vi "ReadIOValues b2g2.vi"(2 "error in":errorcluster, 3 "Output - Cluster b2g2 2":T1 {"TS-5 [°C]" format="%#.2g"; "pHS-1 [pH]" format="%.2g"; "TS-4 [°C]" format="%#.2g"; "FS-2 [l]" format="%.2g"; "FS-1 [l]" format="%.2g"; "DS-1 [bar]" format="%#.2g"; "DFS-1 [l/min]" format="%#.2g"; "FS-3 [l]" format="%.2g"; "DFS-1 [dl]" format="%.0g"}) -> (0 "error out":errorcluster, 1 "Output - Cluster b2g2":T1 {"TS-5 [°C]" format="%#.2g"; "pHS-1 [pH]" format="%.2g"; "TS-4 [°C]" format="%#.2g"; "FS-2 [l]" format="%.2g"; "FS-1 [l]" format="%.2g"; "DS-1 [bar]" format="%#.2g"; "DFS-1 [l/min]" format="%#.2g"; "FS-3 [l]" format="%.2g"; "DFS-1 [dl]" format="%.0g"})   [LabVIEW 2011]
uses:
  Output - Cluster b2g2.ctl
  <vilib>/functionblocks/Counter/Count Up/Count Up.vi
  <vilib>/functionblocks/FB Core/FB Core.xnode
  <vilib>/functionblocks/NI_FunctionBlock Libraries.lvlib
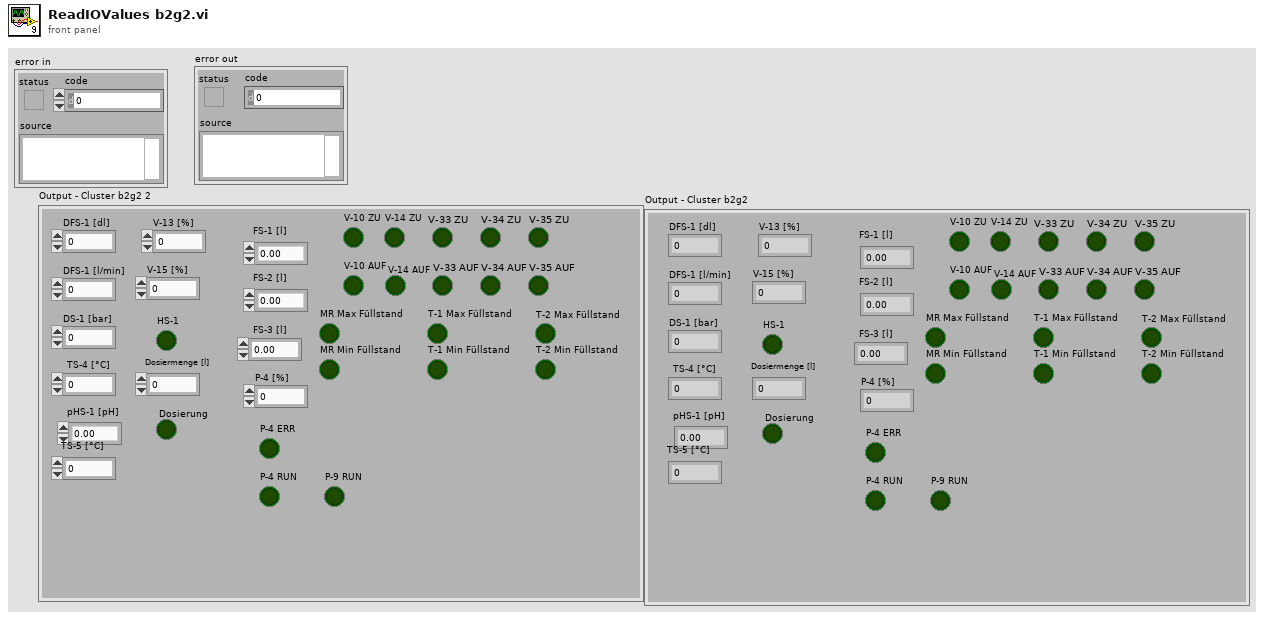
[diagram p1: front panel]
types:
  T1 = typedef "Output - Cluster b2g2.ctl" = cluster{"DFS-1 [dl]":u64, "FS-3 [l]":dbl, "DFS-1 [l/min]":dbl, "DS-1 [bar]":dbl, "V-10 ZU":bool, "V-14 ZU":bool, "FS-1 [l]":dbl, "FS-2 [l]":dbl, "TS-4 [°C]":dbl, "HS-1":bool, "V-13 [%]":u8, "V-15 [%]":u8, "P-4 [%]":u8, "Dosierung":bool, "MR Max Füllstand":bool, "MR Min Füllstand":bool, "Dosiermenge [l]":sgl, "V-14 AUF":bool, "V-10 AUF":bool, "T-1 Max Füllstand":bool, "T-1 Min Füllstand":bool, "T-2 Max Füllstand":bool, "T-2 Min Füllstand":bool, "pHS-1 [pH]":dbl, "P-4 RUN":bool, "V-33 AUF":bool, "V-33 ZU":bool, "V-34 AUF":bool, "V-34 ZU":bool, "P-4 ERR":bool, "TS-5 [°C]":dbl, "V-35 AUF":bool, "V-35 ZU":bool, "P-9 RUN":bool}
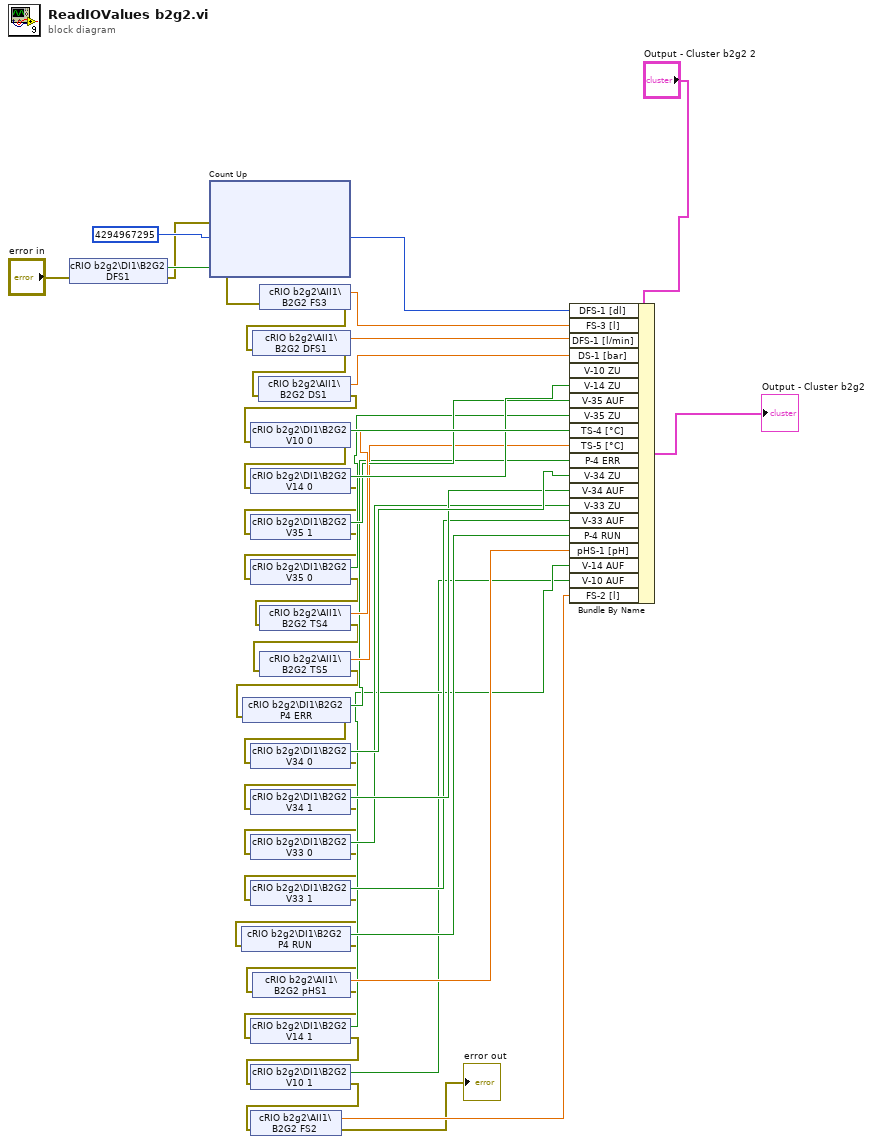
[diagram p0: block diagram]
diagram:
  n1 = shared-variable "cRIO b2g2\\DI1\\B2G2 DFS1"(error in="error in") -> (w40:bool, error out=w23:errorcluster)
  n2 = xnode "Count Up"("error in"=w23, "preset value"=u32 4294967295, "count up"=w40) -> ("error out"=w22:errorcluster, "counter value"=w46:u32)  [unwired: 1 in, 1 out]
  n3 = shared-variable "cRIO b2g2\\AII1\\B2G2 FS3"(error in=w22) -> (w43:dbl, error out=w21:errorcluster)
  n4 = shared-variable "cRIO b2g2\\AII1\\B2G2 DFS1"(error in=w21) -> (w42:dbl, error out=w20:errorcluster)
  n5 = shared-variable "cRIO b2g2\\AII1\\B2G2 DS1"(error in=w20) -> (w41:dbl, error out=w19:errorcluster)
  n6 = shared-variable "cRIO b2g2\\DI1\\B2G2 V10 0"(error in=w19) -> (w39:bool, error out=w18:errorcluster)
  n7 = shared-variable "cRIO b2g2\\DI1\\B2G2 V14 0"(error in=w18) -> (w38:bool, error out=w17:errorcluster)
  n8 = shared-variable "cRIO b2g2\\DI1\\B2G2 V35 1"(error in=w17) -> (w36:bool, error out=w16:errorcluster)
  n9 = shared-variable "cRIO b2g2\\DI1\\B2G2 V35 0"(error in=w16) -> (w35:bool, error out=w15:errorcluster)
  n10 = shared-variable "cRIO b2g2\\AII1\\B2G2 TS4"(error in=w15) -> (w37:dbl, error out=w14:errorcluster)
  n11 = shared-variable "cRIO b2g2\\AII1\\B2G2 TS5"(error in=w14) -> (w34:dbl, error out=w13:errorcluster)
  n12 = shared-variable "cRIO b2g2\\DI1\\B2G2 P4 ERR"(error in=w13) -> (w33:bool, error out=w12:errorcluster)
  n13 = shared-variable "cRIO b2g2\\DI1\\B2G2 V34 0"(error in=w12) -> (w32:bool, error out=w11:errorcluster)
  n14 = shared-variable "cRIO b2g2\\DI1\\B2G2 V34 1"(error in=w11) -> (w31:bool, error out=w10:errorcluster)
  n15 = shared-variable "cRIO b2g2\\DI1\\B2G2 V33 0"(error in=w10) -> (w30:bool, error out=w9:errorcluster)
  n16 = shared-variable "cRIO b2g2\\DI1\\B2G2 V33 1"(error in=w9) -> (w29:bool, error out=w8:errorcluster)
  n17 = shared-variable "cRIO b2g2\\DI1\\B2G2 P4 RUN"(error in=w8) -> (w28:bool, error out=w7:errorcluster)
  n18 = shared-variable "cRIO b2g2\\AII1\\B2G2 pHS1"(error in=w7) -> (w27:dbl, error out=w6:errorcluster)
  n19 = shared-variable "cRIO b2g2\\DI1\\B2G2 V14 1"(error in=w6) -> (w26:bool, error out=w5:errorcluster)
  n20 = shared-variable "cRIO b2g2\\DI1\\B2G2 V10 1"(error in=w5) -> (w25:bool, error out=w2:errorcluster)
  n21 = shared-variable "cRIO b2g2\\AII1\\B2G2 FS2"(error in=w2) -> (w3:dbl, error out=→"error out":errorcluster)
  n22 = Bundle By Name(cluster="Output - Cluster b2g2 2", "DFS-1 [dl]"=w46, "FS-3 [l]"=w43, "DFS-1 [l/min]"=w42, "DS-1 [bar]"=w41, "V-10 ZU"=w39, "V-14 ZU"=w38, "V-35 AUF"=w36, "V-35 ZU"=w35, "TS-4 [°C]"=w37, "TS-5 [°C]"=w34, "P-4 ERR"=w33, "V-34 ZU"=w32, "V-34 AUF"=w31, "V-33 ZU"=w30, "V-33 AUF"=w29, "P-4 RUN"=w28, "pHS-1 [pH]"=w27, "V-14 AUF"=w26, "V-10 AUF"=w25, "FS-2 [l]"=w3) -> (→"Output - Cluster b2g2":T1)
